vi "Channel Properties - Get URL.vi"(8 "error in (no error)":errorcluster, 11 "Channel Ref in":T1 format="%.0x") -> (0 "error out":errorcluster, 2 "Shared Variable URL":string, 3 "Channel Ref out":T1 format="%.0x")   [LabVIEW 2012, in "Shared Variable Custom Device.lvlib"]
uses:
  Shared Variable Custom Device.lvlib
  <vilib>/NI Veristand/Custom Device API/Custom Device Item Ref.ctl
  Shared Variable Globals.vi
  <vilib>/NI Veristand/Custom Device API/Get Item Property (String).vi
  <vilib>/NI Veristand/Custom Device API/Custom Device API.lvlib
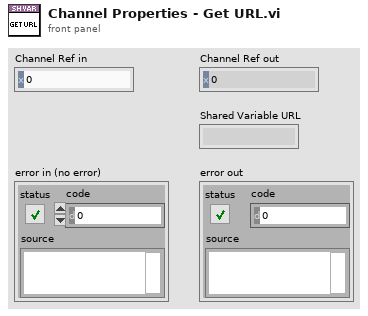
[diagram p1: front panel]
types:
  T1 = typedef "Custom Device API.lvlib/Custom Device Item Ref.ctl" = u64
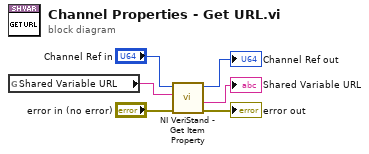
[diagram p0: block diagram]
diagram:
  n1 = global read "Shared Variable Globals.vi" "Shared Variable URL"() -> (w3:string)
  n2 = call-poly <vilib>:"NI VeriStand - Get Item Property.vi"("error in (no error)"="error in (no error)", "Property Name"=w3, "Item Ref in"="Channel Ref in") -> ("error out"=→"error out":errorcluster, "Value"=→"Shared Variable URL":string, "Item Ref out"=→"Channel Ref out":T1)  [unwired: 5 in, 1 out]
